vi "Shift Rows2.vi"(7 "Nb":i32=4, 8 "error in":errorcluster, 10 "State In":u16[][](array[numeric])=[[255, 97, 23, 96], [160, 160, 73, 200], [205, 24, 172, 154], [50, 93, 135, 180]]) -> (0 "error out":errorcluster, 2 "State Out":u16[][](array[numeric]))   [LabVIEW 2013]
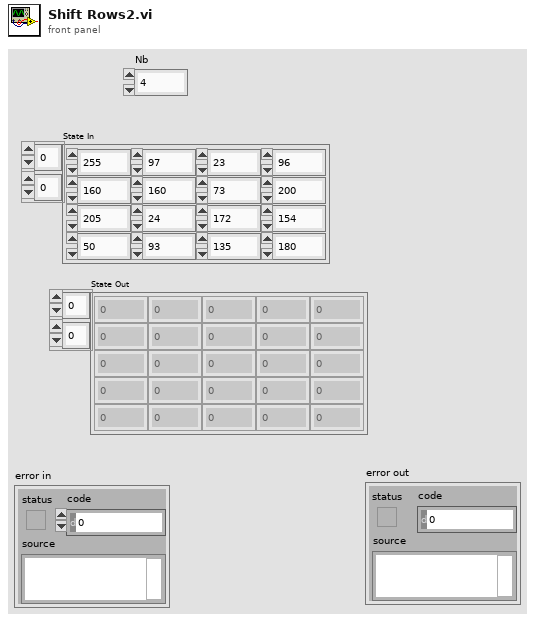
[diagram p1: front panel]
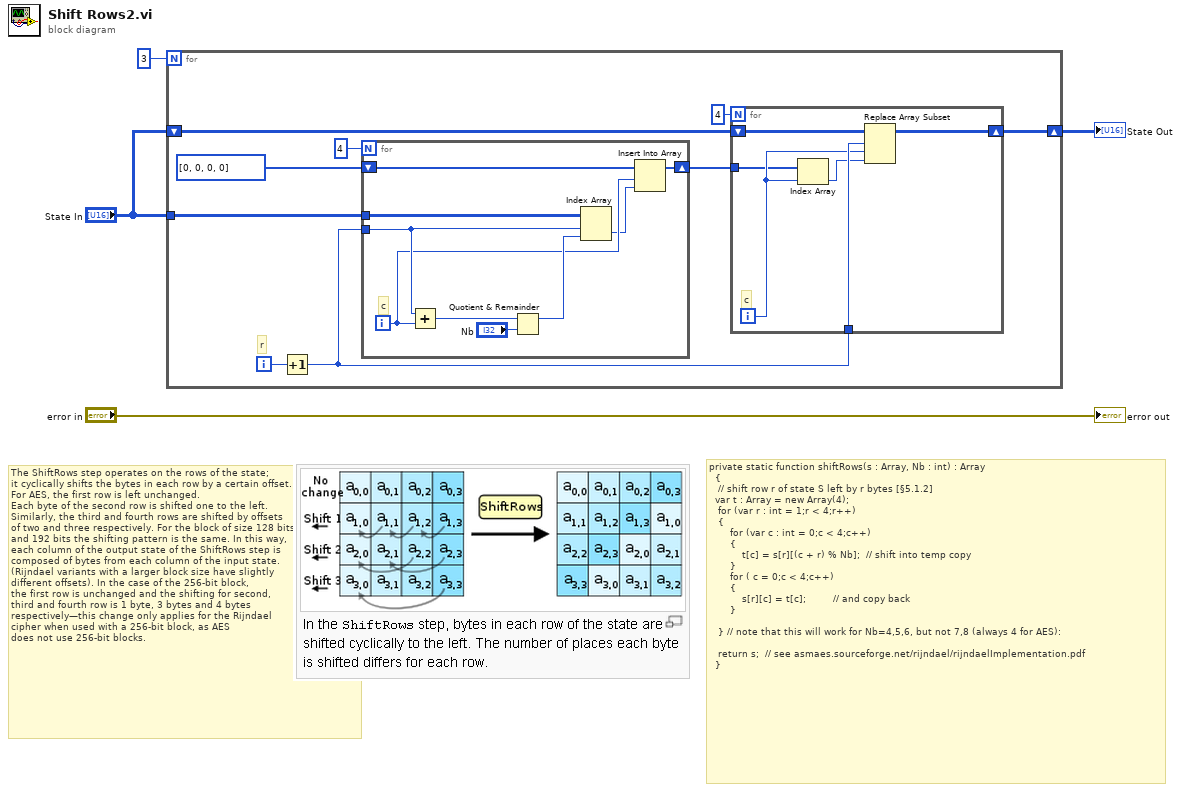
[diagram p0: block diagram]
diagram:
  # "The ShiftRows step operates on the rows of the state; \nit cyclically shifts the bytes in each row by a certain offset. \nFor AES, the first row is left unchanged. \nEach byte of the second row is shifted one to the left. \nSimilarly, the third and fourth rows are shifted by offsets \nof two and three respectively. For the block of size 128 bits \nand 192 bits the shifting pattern is the same. In this way, \neach column of the output state of the ShiftRows step is \ncomposed of bytes from each column of the input state. \n(Rijndael variants with a larger block size have slightly \ndifferent offsets). In the case of the 256-bit block, \nthe first row is unchanged and the shifting for second, \nthird and fourth row is 1 byte, 3 bytes and 4 bytes \nrespectively—this change only applies for the Rijndael \ncipher when used with a 256-bit block, as AES \ndoes not use 256-bit blocks."
  # "private static function shiftRows(s : Array, Nb : int) : Array \n\t\t{    \n\t\t\t// shift row r of state S left by r bytes [§5.1.2]\n\t\tvar t : Array = new Array(4);\n\t\t\tfor (var r : int = 1;r < 4;r++) \n\t\t\t{\n\t\t\t\t   for (var c : int = 0;c < 4;c++) \n\t\t\t\t   {\n\t\t\t\t\t      t[c] = s[r][(c + r) % Nb];  // shift into temp copy\n\t\t\t\t   }\n\t\t\t\t   for ( c = 0;c < 4;c++) \n\t\t\t\t   {\n\t\t\t\t      \ts[r][c] = t[c];         // and copy back\n\t\t\t\t   }\n\t\t\t\t\n\t\t\t} // note that this will work for Nb=4,5,6, but not 7,8 (always 4 for AES):\n\n\t\t\treturn s;  // see asmaes.sourceforge.net/rijndael/rijndaelImplementation.pdf\n\t\t}"
  n1 = for {
    N: 3 -> [_]
    tunnel: "State In" -> [w13]
    shift-right: [w9] -> w2
    shift-left: "State In" -> [w10]
    i -> [w12]
    # "r"
    n2 = Increment(x=w12) -> (x+1=w11:i32)
    n3 = for {
      N: 4 -> [_]
      tunnel: w13 -> [w28]
      tunnel: w11 -> [w24]
      shift-right: [w20] -> w7
      shift-left: i32[] [0, 0, 0, 0] ("t[c]") -> [w21]
      i -> [w23]
      # "c"
      n4 = Add(x=w24, y=w23) -> (x+y=w27:i32)
      n5 = Quotient & Remainder(x=w27, y="Nb") -> (x-y*floor(x/y)=w25:i32)  [unwired: 1 out]
      n6 = Index Array(array=w28, index (row)=w24, index (col)=w25) -> (element=w22:u16)
      n7 = Insert Into Array(array=w21, index=w23, new element=w22) -> (w20:i32[])
    }
    n8 = for {
      N: 4 -> [_]
      tunnel: w11 -> [w19]
      shift-right: [w15] -> w9
      shift-left: w10 -> [w16]
      tunnel: w7 -> [w14]
      i -> [w18]
      # "c"
      n9 = Index Array(array=w14, index=w18) -> (element=w17:i32)
      n10 = Replace Array Subset(array=w16, new element=w17, index (row)=w19, index (col)=w18) -> (w15:u16[][])
    }
  }
  "State Out" <- w2
  "error out" <- "error in"
